vi "JSON Parse Info.vi"(0 "JSON":string, 11 "error in (no error)":errorcluster) -> (4 "results-JSON":string caption="results-JSON string", 6 "ID":i32, 8 "returned command":string, 10 "error string (if existing)":string, 15 "error out":errorcluster)   [LabVIEW 2023, in "Communicator.lvclass"]
uses:
  Communicator.lvclass
panel:
  # "Connector Pane"
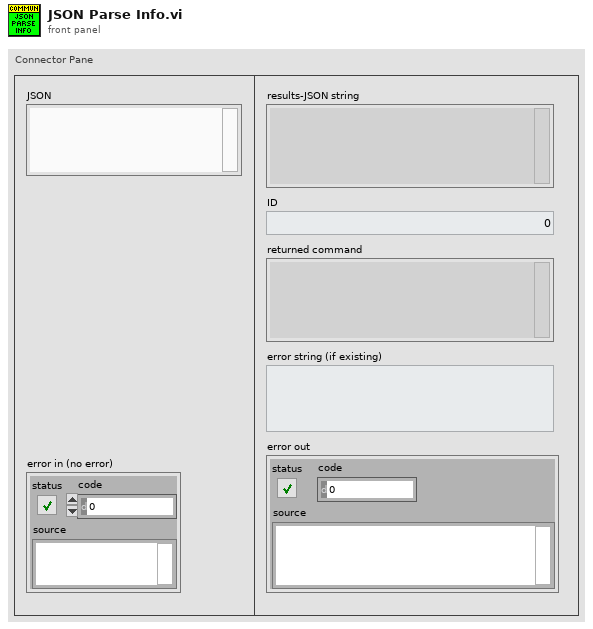
[diagram p1: front panel]
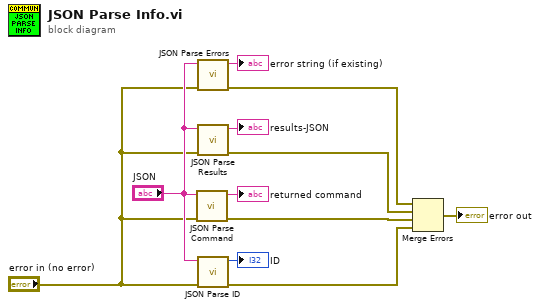
[diagram p0: block diagram]
diagram:
  n1 = call "JSON Parse Command.vi"("error in (no error)"="error in (no error)", "JSON command"="JSON") -> ("error out"=w2:errorcluster, "returned command"=→"returned command":string)  [unwired: 7 in, 1 out]
  n2 = call "JSON Parse Errors.vi"("error in (no error)"="error in (no error)", "JSON command"="JSON") -> ("error out"=w4:errorcluster, "error string (if existing)"=→"error string (if existing)":string)  [unwired: 7 in, 1 out]
  n3 = call "JSON Parse Results.vi"("error in (no error)"="error in (no error)", "JSON"="JSON") -> ("error out"=w3:errorcluster, "results-JSON"=→"results-JSON":string)  [unwired: 7 in, 1 out]
  n4 = call "JSON Parse ID.vi"("error in (no error)"="error in (no error)", "JSON"="JSON") -> ("error out"=w1:errorcluster, "ID"=→"ID":i32)  [unwired: 7 in, 1 out]
  n5 = Merge Errors(w4, w3, w2, w1) -> (→"error out":errorcluster)
